vi "EEG_Main.vi"() -> ()   [LabVIEW 2026]
uses:
  <vilib>/httpClient/ClientHandle.ctl
  <vilib>/Analysis/baseanly.llb/Mean (DBL).vi
  <vilib>/Analysis/2dsp.llb/Power Spectrum (DBL).vi
  <vilib>/Analysis/5stat.llb/RMS (DBL).vi
  <vilib>/Utility/file.llb/Read Delimited Spreadsheet (DBL).vi
  <vilib>/httpClient/POSTBuffer.vi
  <vilib>/httpClient/LabVIEWHTTPClient.lvlib
  <vilib>/Analysis/NI_AALPro.lvlib
  <vilib>/Analysis/NI_AALBase.lvlib
panel:
  out "Response Body":string
  out "Response Headers":string
  out "client handle out":T1
  out "http_handle":T1
  out "json_a_envoyer":string
  out "json_final":string
  out "energie_rms":dbl format="%0.2f"
  out "segment_id":dbl
  out "label_reel":string
  out "est_crise":bool
  out "y_valeur":dbl
  out "spectre":dbl[](array[numeric])
  out "log2(x)":dbl
  out "frequence_dominante_hz":dbl
  out "index_pic":i32
  out "entropie_spectrale":dbl
  out "somme_p_log_p":dbl
  out "p_log_p":dbl[](array[numeric])
  out "log2_p":dbl[](array[numeric])
  out "sum_normalise":dbl
  out "verif_spectre_avant_div":dbl[](array[numeric])
  out "p_epsilon":dbl[](array[numeric])
  out "p_normalise":dbl[](array[numeric])
  out "somme_spectre":dbl
  out "Power Spectrum":dbl[](array[numeric])
  out "signal_centre":dbl[](array[numeric])
  out "signal_pur":dbl[](array[numeric])
  out "segment_test":dbl[](array[numeric])
  out "all rows 2":dbl[][](array[numeric])
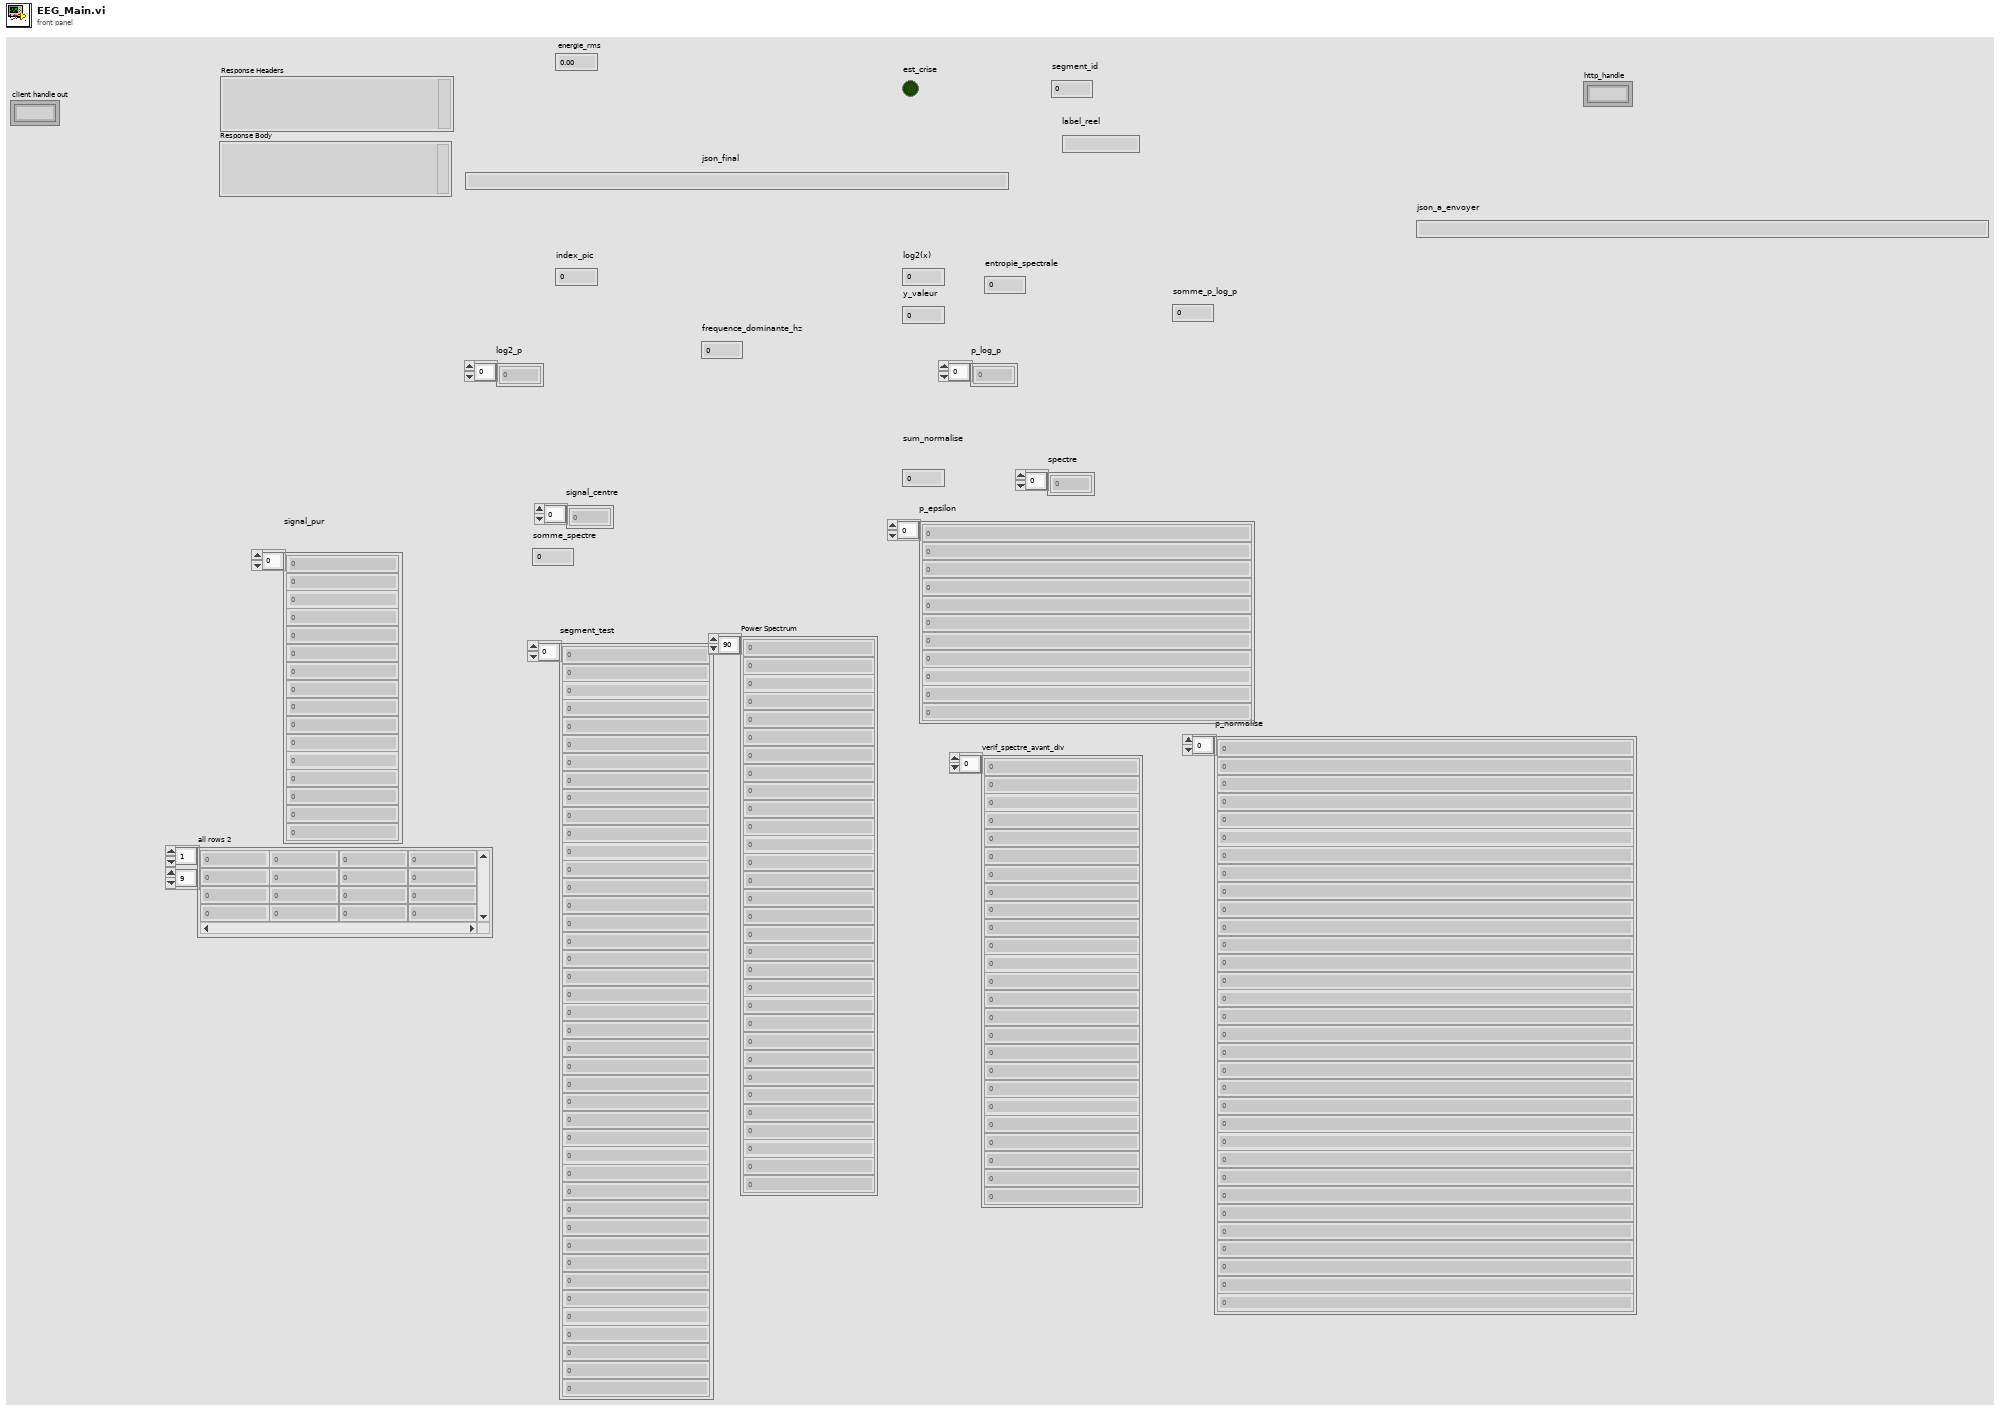
[diagram p1: front panel]
types:
  T1 = typedef "LabVIEWHTTPClient.lvlib/ClientHandle.ctl" = refnum<k1>
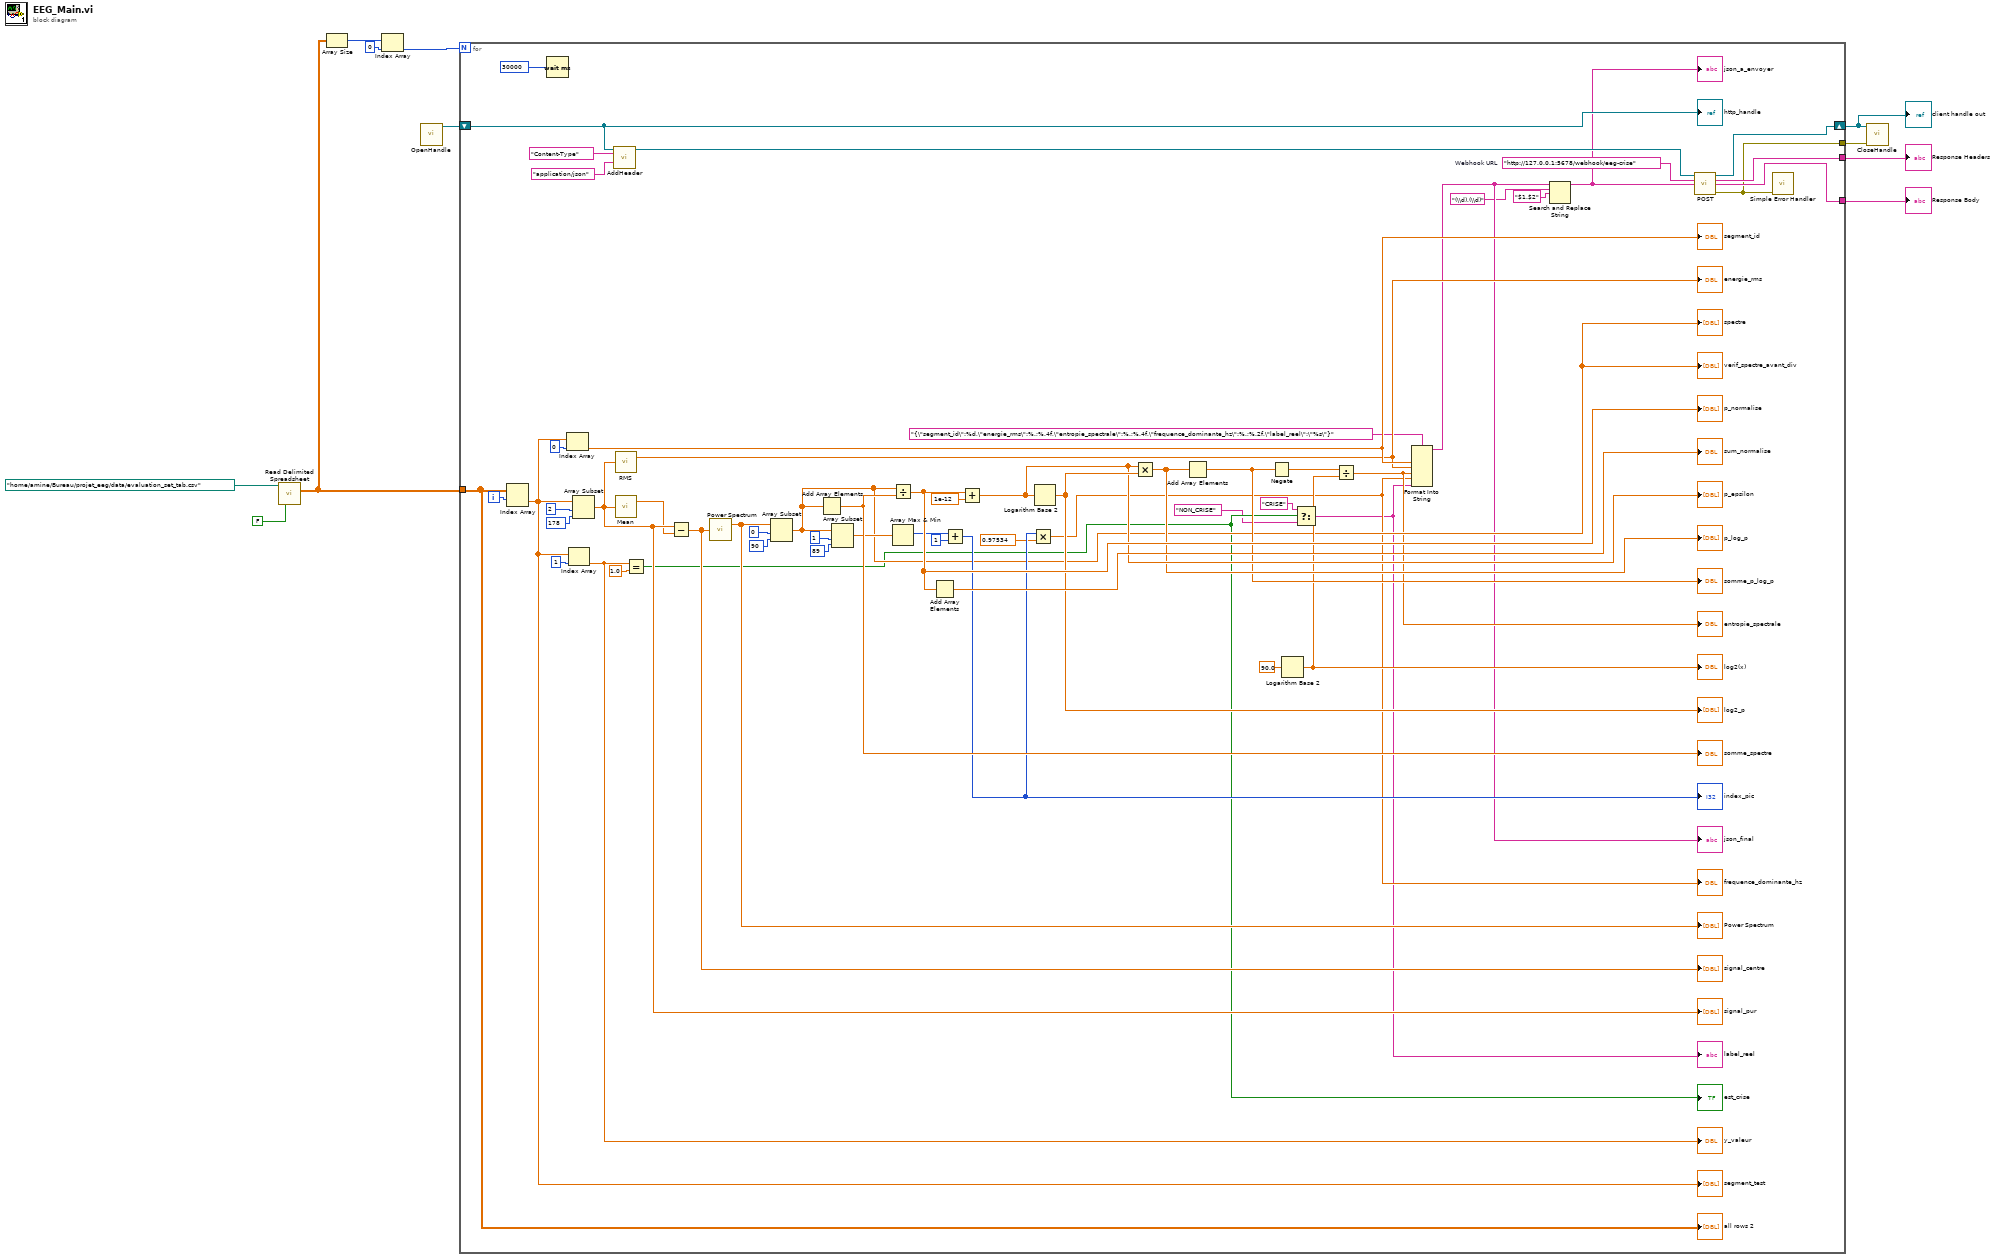
[diagram p0: block diagram]
diagram:
  n1 = call-poly <vilib>:"Read Delimited Spreadsheet.vi"("file path (dialog if empty)"=path "/home/amine/Bureau/projet_eeg/data/evaluation_set_tab.csv", "transpose? (F)"=FALSE) -> ("all rows"=w4:dbl[][])  [unwired: 8 in, 5 out]
  n2 = Array Size(array=w4) -> (size(s)=w3:i32[])
  n3 = Index Array(array=w3, index=0) -> (element=w1:i32)
  n4 = call <vilib>:"OpenHandle.vi"() -> ("client handle out"=w11:T1)  [unwired: 14 in, 1 out]
  n5 = for {
    N: w1 -> [_]
    tunnel: [w18] -> w10
    tunnel: [w17] -> w9
    tunnel: [w12] -> w8
    shift-right: [w16] -> w7
    shift-left: w11 -> [w24]
    tunnel: w4 -> [w14]
    i -> [w15]
    w22 = "http://127.0.0.1:5678/webhook/eeg-crise"  # Webhook URL
    n6 = Index Array(array=w14, index (row)=w15) -> (element=w34:dbl[])  [unwired: 1 in]
    "segment_test" <- w34
    n7 = Wait (ms)(milliseconds to wait=u32 30000) -> ()  [unwired: 1 out]
    n8 = Index Array(array=w34, index=0) -> (element=w33:dbl)
    "segment_id" <- w33
    n9 = Index Array(array=w34, index=1) -> (element=w40:dbl)
    "y_valeur" <- w40
    n10 = Array Subset(array=w34, index=2, length=178) -> (w66:dbl[])
    "signal_pur" <- w66
    n11 = call <vilib>:"AddHeader.vi"("client handle"=w24, "header"="Content-Type", "value"="application/json") -> ("client handle out"=w23:T1)  [unwired: 11 in, 1 out]
    n12 = call-poly <vilib>:"RMS.vi"("X"=w66) -> ("rms value"=w32:dbl)  [unwired: 1 out]
    "energie_rms" <- w32
    n13 = call-poly <vilib>:"Mean.vi"("X"=w66) -> ("mean"=w65:dbl)  [unwired: 1 out]
    n14 = Equal?(x=w40, y=1.0) -> (x = y?=w38:bool)
    "est_crise" <- w38
    n15 = Subtract(x=w66, y=w65) -> (x-y=w64:dbl[])
    "signal_centre" <- w64
    n16 = call-poly <vilib>:"Power Spectrum.vi"("X"=w64) -> ("Power Spectrum"=w45:dbl[])  [unwired: 1 out]
    "Power Spectrum" <- w45
    n17 = Array Subset(array=w45, index=0, length=90) -> (w42:dbl[])
    "verif_spectre_avant_div" <- w42
    "spectre" <- w42
    n18 = Add Array Elements(numeric array=w42) -> (sum=w63:dbl)
    "somme_spectre" <- w63
    n19 = Array Subset(array=w42, index=1, length=89) -> (w49:dbl[])
    n20 = Divide(x=w42, y=w63) -> (x/y=w60:dbl[])
    "p_normalise" <- w60
    n21 = Array Max & Min(array=w49) -> (max index (indices)=w50:i32)  [unwired: 3 out]
    n22 = Add Array Elements(numeric array=w60) -> (sum=→"sum_normalise":dbl)
    n23 = Add(x=w50, y=1) -> (x+y=w48:i32)
    "index_pic" <- w48
    n24 = Add(x=w60, y=1e-12) -> (x+y=w58:dbl[])
    "p_epsilon" <- w58
    n25 = Multiply(x=w48, y=0.97534) -> (x*y=w30:dbl)
    "frequence_dominante_hz" <- w30
    n26 = Logarithm Base 2(1:w58) -> (0:w59:dbl[])
    "log2_p" <- w59
    n27 = Multiply(x=w58, y=w59) -> (x*y=w57:dbl[])
    "p_log_p" <- w57
    n28 = Add Array Elements(numeric array=w57) -> (sum=w56:dbl)
    "somme_p_log_p" <- w56
    n29 = Negate(x=w56) -> (-x=w55:dbl)
    n30 = Logarithm Base 2(1:90.0 ("x")) -> (0:w46:dbl)
    "log2(x)" <- w46
    n31 = Select(t="CRISE", s=w38, f="NON_CRISE") -> (s? t:f=w29:string)
    "label_reel" <- w29
    n32 = Divide(x=w55, y=w46) -> (x/y=w31:dbl)
    "entropie_spectrale" <- w31
    n33 = Format Into String(format string="{\"segment_id\":%d,\"energie_rms\":%.;%.4f,\"entropie_spectrale\":%.;%.4f,\"frequence_dominante_hz\":%.;%.2f,\"label_reel\":\"%s\"}", w33, w32, w31, w30, w29) -> (resulting string=w27:string)  [unwired: 2 in, 1 out]
    "json_final" <- w27
    n34 = Search and Replace String(input string=w27, search string="(\\d),(\\d)", replace string="$1.$2") -> (result string=w19:string)  [unwired: 5 in, 3 out]
    "json_a_envoyer" <- w19
    n35 = call-poly <vilib>:"POST.vi"("client handle"=w23, "url"=w22, "buffer"=w19) -> ("client handle out"=w16:T1, "headers"=w18:string, "body"=w17:string, "error out"=w12:errorcluster)  [unwired: 9 in]
    n36 = call <vilib>:"Simple Error Handler.vi"("error in (no error)"=w12) -> ()  [unwired: 4 in, 5 out]
    "all rows 2" <- w14
    "http_handle" <- w24
  }
  "client handle out" <- w7
  "Response Headers" <- w10
  "Response Body" <- w9
  n37 = call <vilib>:"CloseHandle.vi"("client handle"=w7, "error in (no error)"=w8) -> ()  [unwired: 13 in, 1 out]
